vi "FGV Lebt cRIO.vi"() -> (1 "lebt cRIO?":bool)   [LabVIEW 2020, in "Kommunikation mit cRIO.lvlib"]
uses:
  Kommunikation mit cRIO.lvlib
  Stoerungen/Stoerungen Messgeraet/Aktionen Kommunikation Stoerung.ctl
  Seiten/System Einstellungen V2/Aktioen FGV System.ctl
  Stoerungen/Stoerungen.lvlib
  Seiten/System Einstellungen V2/System Einstellungen V2.lvlib
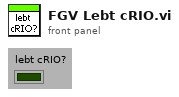
[diagram p1: front panel]
types:
  T1 = typedef "System Einstellungen V2.lvlib/Aktioen FGV System.ctl" = enum16{"lesen", "laden", "speichern", "Optionen schreiben", "Zeitstempel", "Reset BMP", "Reset SQP", "Wartung", "Werkseinstellung"}
  T2 = typedef "Stoerungen.lvlib/Aktionen Kommunikation Stoerung.ctl" = enum16{"lesen", "init", "FT-IR Komm", "FT-IR Betriebsart", "FT-IR Hintergrund", "cRIO Komm", "PNS Komm", "Dichtheitstest", "Life Bit", "FTIR Komm AK", "PMA Komm", "FID Komm", "PMA Cal", "FID Ch4 Cal", "FID THC Cal", "Cal Timeout", "VFS 1 Komm", "VFS 2 Komm", "VFS 3 Komm", "VFS 4 Komm", "TRE 08 Komm", "CG-Test vorzeitig", "CG-Test Span 1", "CG-Test Span 2", "CG-Test Span 3", "CG-Test Messgas", "CG-Test löschen", "Test", "Amium AK", "AK Recept konfig", "AK Name konfig", "AK EKFG konfig"}
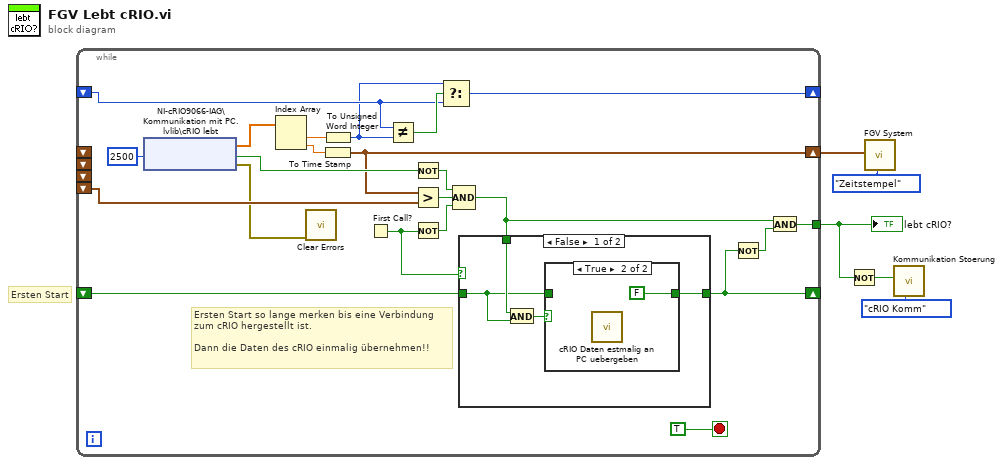
[diagram p0: block diagram]
diagram:
  # "Ersten Start"
  n1 = while {
    shift-right: [w26] -> _
    shift-left: _ -> [w24]
    shift-right: [w6] -> w1
    shift-left: _ -> [_]
    shift-left: _ -> [_]
    shift-left: _ -> [_]
    shift-left: _ -> [w21]
    tunnel: [w11] -> w4
    shift-right: [w12] -> _
    shift-left: _ -> [w16]
    stop <- TRUE stop-if-true
    # "Ersten Start so lange merken bis eine Verbindung\nzum cRIO hergestellt ist.\n\nDann die Daten des cRIO einmalig übernehmen!!"
    n2 = shared-variable "NI-cRIO9066-IAG\\Kommunikation mit PC.lvlib\\cRIO lebt"(2500 ("Timeout in ms(0)")) -> (w8:dbl[], error out=w17:errorcluster, w20:bool)  [unwired: 1 out]
    n3 = Index Array(array=w8) -> (element #1=w9:dbl, element #2=w10:dbl)  [unwired: 2 in]
    n4 = call <vilib>:"Clear Errors.vi"("error in (no error)"=w17) -> ()  [unwired: 1 in, 6 out]
    n5 = To Unsigned Word Integer(number=w9) -> (unsigned 16bit integer=w7:u16)
    n6 = To Time Stamp(1:w10) -> (0:w6:timestamp)
    n7 = First Call?() -> (First Call?: T/F=w15:bool)
    n8 = Not Equal?(x=w24, y=w7) -> (x != y?=w25:bool)
    n9 = Not(x=w20) -> (.not. x?=w19:bool)
    n10 = Greater?(x=w6, y=w21) -> (0:w22:bool)
    n11 = Not(x=w15) -> (.not. x?=w23:bool)
    n12 = Select(t=w7, s=w25, f=w24) -> (s? t:f=w26:u16)
    n13 = Compound Arithmetic op=AND(w19, w22, w23) -> (w14:bool)
    n14 = case shown="False" w15 {
      selector: w15 -> [_ w34]
      tunnel: [w31 w34] -> w12
      tunnel: w16 -> [w28 _]
      tunnel: w14 -> [w29 _]
      frame False {
        n15 = And(x=w29, y=w28) -> (x .and. y?=w30:bool)
        n16 = case shown="True" w30 {
          tunnel: [w32 FALSE] -> w31
          tunnel: w28 -> [w32 _]
          frame False {
          }
          frame True {
            n17 = call "cRIO Daten estmalig an PC uebergeben.vi"() -> ()  [unwired: 11 in, 1 out]
          }
        }
      }
      frame True {
      }
    }
    n18 = Not(x=w12) -> (.not. x?=w13:bool)
    n19 = And(x=w14, y=w13) -> (x .and. y?=w11:bool)
  }
  "lebt cRIO?" <- w4
  n20 = Not(x=w4) -> (.not. x?=w3:bool)
  n21 = call "FGV System.vi"("Zeitstempel"=w1, "Aktionen"=Aktioen_FGV_System."Zeitstempel") -> ()  [unwired: 11 in, 7 out]
  n22 = call "Kommunikation Stoerung.vi"("Aktionen"=Aktionen_Kommunikation_Stoerung."cRIO Komm", "ERROR"=w3) -> ()  [unwired: 9 in, 1 out]
